vi "DSF.Engine.Builder.Buffer.Get Tx Transfer.vi"(8 "error in (no error)":errorcluster, 10 "build/parse command":T1, 11 "Builder in":refnum<class "DSF.Engine.Builder.lvclass">) -> (0 "error out":errorcluster, 2 "Transfer":refnum<class "DSF.Engine.Transfer.lvclass">, 3 "Builder out":refnum<class "DSF.Engine.Builder.lvclass">)   [LabVIEW 2017, in "DSF.Engine.lvlib" / "DSF.Engine.Builder.lvclass"]
uses:
  DSF.Engine.Builder.lvclass
  DSF.Engine.Builder.Command.Build-Parse.ctl
  Transfer/DSF.Engine.Transfer.lvclass
  DSF.Engine.Builder.lvclass/DSF.Engine.Builder.ctl
  Plugin/Plugin.lvclass/Plugin.ctl
  Transfer/DSF.Engine.Transfer Group.lvclass/DSF.Engine.Transfer Group.ctl
  Plugin/Plugin.lvclass
  Transfer/DSF.Engine.Transfer Group.lvclass
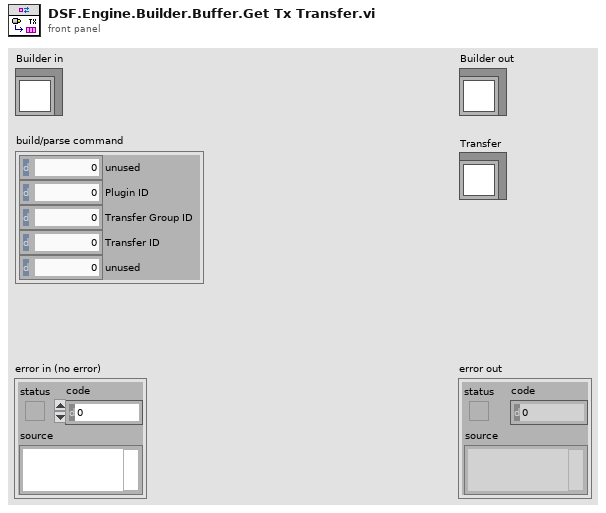
[diagram p1: front panel]
types:
  T1 = typedef "DSF.Engine.lvlib/DSF.Engine.Builder.lvclass/DSF.Engine.Builder.Command.Build-Parse.ctl" = cluster{"unused":u8, "Plugin ID":i32, "Transfer Group ID":i32, "Transfer ID":i32, "unused":i32}
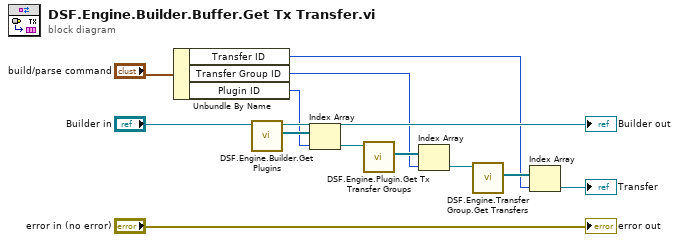
[diagram p0: block diagram]
diagram:
  n1 = Unbundle By Name("build/parse command") -> ("Transfer ID"=w3:i32, "Transfer Group ID"=w2:i32, "Plugin ID"=w1:i32)
  n2 = call "DSF.Engine.Builder.Get Plugins.vi"("Builder in"="Builder in") -> ("Plugins"=w12:refnum<class "Plugin.lvclass">[], "Builder out"=→"Builder out":refnum<class "DSF.Engine.Builder.lvclass">)  [unwired: 9 in]
  n3 = Index Array(array=w12, index=w1) -> (element=w11:refnum<class "Plugin.lvclass">)
  n4 = call "DSF.Engine.Plugin.Get Tx Transfer Groups.vi"("Plugin in"=w11) -> ("Tx Transfer Groups"=w10:refnum<class "DSF.Engine.Transfer Group.lvclass">[])  [unwired: 9 in, 1 out]
  n5 = Index Array(array=w10, index=w2) -> (element=w9:refnum<class "DSF.Engine.Transfer Group.lvclass">)
  n6 = call "DSF.Engine.Transfer Group.Get Transfers.vi"("Transfer Group in"=w9) -> ("Transfers"=w8:refnum<class "DSF.Engine.Transfer.lvclass">[])  [unwired: 9 in, 1 out]
  n7 = Index Array(array=w8, index=w3) -> (element=→"Transfer":refnum<class "DSF.Engine.Transfer.lvclass">)
  "error out" <- "error in (no error)"
